vi "红外遥控解码实验.vi"   [LabVIEW 2011]
uses:
  <vilib>/STM32_DriverVI_Interface_F4/LCD/Brush Color_Index_F4.ctl
  <vilib>/STM32_DriverVI_Interface_F4/LCD/Font_Size_F4.ctl
  <vilib>/STM32_DriverVI_Interface_F4/LCD/Show_Mode_F4.ctl
  <vilib>/STM32_DriverVI_Interface_F4/LCD/LCD_Init_F4.vi
  <vilib>/STM32_DriverVI_Interface_F4/Infrared/Infrared-Globe_F4.vi
types:
  T1 = typedef "Show_Mode_F4.ctl" = enum8{"非叠加显示", "叠加显示"}
  T2 = typedef "Font_Size_F4.ctl" = enum8{"Small_Font（12）", "Big_Font（16）"}
  T3 = typedef "Brush Color_Index_F4.ctl" = enum8{"White", "Black", "Blue", "Green_Blue", "Red", "Magenta（品红）", "Green", "Cyan（青色）", "Yellow", "Brown", "Brown_Red", "Gray", "Dark_Blue", "Light_Blue", "Gray_Blue", "Light_Green", "Light_Gray", "Light_Gray_Blue", "Light_Brown_Blue"}
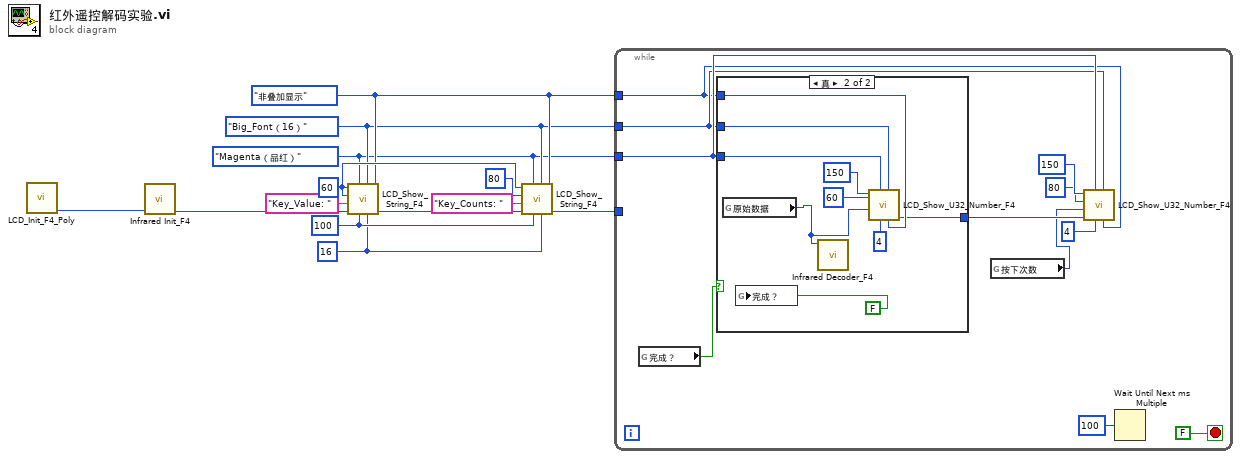
[diagram p0: block diagram]
diagram:
  w1 = u16 16 ("Height")
  w2 = u16 100 ("Width")
  w6 = Show_Mode_F4."非叠加显示" ("Show_Mode")
  w5 = Font_Size_F4."Big_Font（16）" ("Font_Size")
  w4 = Brush_Color_Index_F4."Magenta（品红）" ("Brush Color")
  w10 = u16 60 ("X_Position")
  n1 = call-poly <vilib>:"LCD_Init_F4_Poly.vi"() -> ("err_out"=w13:u8)  [unwired: 10 in, 1 out]
  n2 = call <vilib>:"Infrared Init_F4.vi"("err_in"=w13) -> ("err_out"=w12:u8)  [unwired: 10 in]
  n3 = call <vilib>:"LCD_Show_String_F4.vi"("Show_Mode"=w6, "Height"=w1, "Font_Size"=w5, "Width"=w2, "Brush Color"=w4, "err_in"=w12, "String"="Key_Value: ", "Y_Position"=w10, "X_Position"=w10) -> ("err_out"=w11:u8)  [unwired: 2 in]
  n4 = call <vilib>:"LCD_Show_String_F4.vi"("Show_Mode"=w6, "Height"=w1, "Font_Size"=w5, "Width"=w2, "Brush Color"=w4, "err_in"=w11, "String"="Key_Counts: ", "Y_Position"=u16 80, "X_Position"=w10) -> ("err_out"=w3:u8)  [unwired: 2 in]
  n5 = while {
    tunnel: w6 -> [w19]
    tunnel: w5 -> [w20]
    tunnel: w4 -> [w21]
    tunnel: w3 -> [_]
    stop <- FALSE stop-if-true
    n6 = global read "Infrared-Globe_F4.vi" "完成？"() -> (w14:bool)
    n7 = case shown="真" w14 {
      tunnel: w21 -> [_ w33]
      tunnel: w20 -> [_ w32]
      tunnel: w19 -> [_ w31]
      tunnel: [_ w27] -> w22
      frame False {
      }
      frame True {
        n8 = global read "Infrared-Globe_F4.vi" "原始数据"() -> (w26:u32)
        n9 = global write "Infrared-Globe_F4.vi" "完成？"(FALSE ("完成？")) -> ()
        n10 = call <vilib>:"Infrared Decoder_F4.vi"("Origin_Data[U32]"=w26) -> ()  [unwired: 9 in, 2 out]
        n11 = call <vilib>:"LCD_Show_U32_Number_F4.vi"("Show_Mode"=w31, "Font_Size"=w32, "Len"=u16 4, "Brush Color"=w33, "U32 Number"=w26, "Y_Position"=u16 60, "X_Position"=u16 150) -> ("err_out"=w27:u8)  [unwired: 4 in]
      }
    }
    n12 = global read "Infrared-Globe_F4.vi" "按下次数"() -> (w15:u8)
    n13 = call <vilib>:"LCD_Show_U32_Number_F4.vi"("Show_Mode"=w19, "Font_Size"=w20, "Len"=u16 4, "Brush Color"=w21, "err_in"=w22, "U32 Number"=w15, "Y_Position"=u16 80, "X_Position"=u16 150) -> ()  [unwired: 3 in, 1 out]
    n14 = Wait Until Next ms Multiple(millisecond multiple=u32 100 ("毫秒倍数")) -> ()  [unwired: 1 out]
  }
